vi "DriveExecuteTestFeedFoward.vi"(8 "error in (no error)":errorcluster) -> (0 "error out":errorcluster)   [LabVIEW 2020]
doc: "Execute and test/tune feed foward for Drive\n\nClosed control loop for drive\n\ninput: \n error in (cluster)\n\noutput:\n error out (cluster)"
uses:
  <vilib>/Rock Robotics/WPI/ThirdParty/Phoenix-LabVIEW/Motor Controller/Controls/CTRE_Phoenix_MotorControl_ControlMode.ctl
  <vilib>/Rock Robotics/WPI/ThirdParty/JAS_Junk/TrajLib/VI/Util_GetTime_U32.vi
  <vilib>/Rock Robotics/WPI/ThirdParty/JAS_Junk/TrajLib/SlewRateLimiter_New.vi
  <vilib>/Rock Robotics/WPI/ThirdParty/JAS_Junk/TrajLib/SlewRateLimiter_Reset.vi
  <vilib>/Rock Robotics/WPI/ThirdParty/JAS_Junk/TrajLib/SlewRateLimiter_Calculate.vi
  <vilib>/Rock Robotics/WPI/ThirdParty/JAS_Junk/TrajLib/SlewRateLimiter_SetRate.vi
  <vilib>/Rock Robotics/SystemInterfaces/Utilities/FPGA_UtilitiesRead LocalTime.vi
  <vilib>/Rock Robotics/WPI/ThirdParty/JAS_Junk/TrajLib/VI/Util_GetTime_U64.vi
  DriveGlobal.vi
  <vilib>/Rock Robotics/WPI/ThirdParty/Phoenix-LabVIEW/Motor Controller/Get/CTRE_Phoenix_MotorController_GetSelectedSensorData.vi
  <vilib>/Rock Robotics/WPI/ThirdParty/JAS_Junk/TrajLib/Trajectory_Library.lvlib
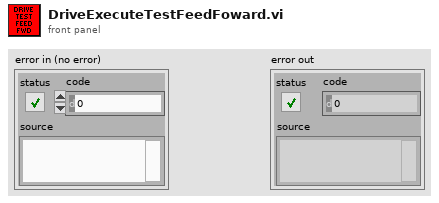
[diagram p1: front panel]
types:
  T1 = typedef "CTRE_Phoenix_MotorControl_ControlMode.ctl" = u16
  T2 = typedef "WPI_MotorControlDeviceRef.ctl" = cluster{"DeviceStatus":errorcluster, "Type":T3, "PWM":cluster{"PWM Channel":T4, "DeadBand":T5}, "CAN":cluster{"Device Number":u8, "SetOutput VI Ref":variant, "GetOutput VI Ref":variant, "Enable VI Ref":variant, "Disable VI Ref":variant, "Data":variant}, "Invert":bool, "DIO PWM":cluster{"PWM \"Enable\" Channel":T4, "DIOChannel":T6, "PWM Rate":dbl}}
  T3 = typedef "WPI_MotorControlType.ctl" = enum16{"PWM", "CAN", "DIO PWM"}
  T4 = typedef "FPGA_DIOPWMChannel.ctl" = enum8{"PWM 0", "PWM 1", "PWM 2", "PWM 3", "PWM 4", "PWM 5", "PWM 6", "PWM 7", "PWM 8", "PWM 9", "PWM MXP 0", "PWM MXP 1", "PWM MXP 2", "PWM MXP 3", "PWM MXP 4", "PWM MXP 5", "PWM MXP 6", "PWM MXP 7", "PWM MXP 8", "PWM MXP 9", "Invalid"}
  T5 = typedef "WPI_PWMDeadband.ctl" = cluster{"Name":string, "maxPositivePwm":i32, "minPositivePwm":i32, "centerPwm":i32, "maxNegativePwm":i32, "minNegativePwm":i32, "angularRange":u16}
  T6 = typedef "FPGA_DIOChannel.ctl" = enum8{"DIO 0", "DIO 1", "DIO 2", "DIO 3", "DIO 4", "DIO 5", "DIO 6", "DIO 7", "DIO 8", "DIO 9", "DIO MXP 0", "DIO MXP 1", "DIO MXP 2", "DIO MXP 3", "DIO MXP 4", "DIO MXP 5", "DIO MXP 6", "DIO MXP 7", "DIO MXP 8", "DIO MXP 9", "DIO MXP 10", "DIO MXP 11", "DIO MXP 12", "DIO MXP 13", "DIO MXP 14", "DIO MXP 15", "SPI Port CS1", "SPI Port CS2", "SPI Port CS3", "SPI Port MISO", "SPI Port MOSI", "Invalid"}
  T7 = typedef "ADIS16470 Device Reference.ctl" = cluster{"DevStatus":errorcluster, "Hardware Config":T8, "Calibration Complete":refnum<notifier>, "Status Reference":refnum<data-value>, "Data Reference":refnum<data-value>, "Sychronous Process VI":T11, "Cmd FIFO":refnum<k33>, "Source":T12, "Data FIFO":refnum<k33>, "Calibration Time (ms)":u32, "Data Reference":refnum<data-value>}
  T8 = typedef "ADIS16470 Hardware Configuration.ctl" = cluster{"SPI Clock Rate (Hz)":dbl, "IMU SPI Mode (3)":T9, "IMU Reset Pin":T6, "IMU SPI Bus":T10, "IMU Data Ready Pin":T6, "Stall Config":cluster{"Pow2BytesPerRead":u8, "StallTicks":u16, "CsToSclkTicks":u8}}
  T9 = typedef "WPI_SPIMode.ctl" = enum16{"Mode 0 (Clk Idle Low,Sample on Leading)", "Mode 1 (Clk Idle Low,Sample on Trailing)", "Mode 2 (Clk Idle High,Sample on Leading)", "Mode 3 (Clk Idle High,Sample on Trailing)"}
  T10 = typedef "spi_bus.ctl" = enum16{"SPI On-Board, CS0", "SPI On-Board, CS1", "SPI On-Board, CS2", "SPI On-Board, CS3", "SPI MXP", "Invalid"}
  T11 = typedef "ADIS16470 Process.ctl" = refnum<vi>
  T12 = typedef "FPGA_CounterEncoderSourceConvertionLVSourceType.ctl" = cluster{"DevStatus":errorcluster, "AnalogTriggerMode?":bool, "DigitalMode":cluster{"DIO Channel":T13}, "AnalogTriggerMode":cluster{"AnalogTriggerIndex":T14, "OutputType":T15}}
  T13 = typedef "FPGA_DIODigitalSourceChannel.ctl" = enum8{"DIO 0", "DIO 1", "DIO 2", "DIO 3", "DIO 4", "DIO 5", "DIO 6", "DIO 7", "DIO 8", "DIO 9", "DIO MXP 0", "DIO MXP 1", "DIO MXP 2", "DIO MXP 3", "DIO MXP 4", "DIO MXP 5", "DIO MXP 6", "DIO MXP 7", "DIO MXP 8", "DIO MXP 9", "DIO MXP 10", "DIO MXP 11", "DIO MXP 12", "DIO MXP 13", "DIO MXP 14", "DIO MXP 15", "SPI Port CS1", "SPI Port CS2", "SPI Port CS3", "SPI Port MISO", "SPI Port MOSI", "Disabled"}
  T14 = typedef "FPGA_AnalogTriggerIndex.ctl" = enum8{"Trig 0", "Trig 1", "Trig 2", "Trig 3", "Trig 4", "Trig 5", "Trig 6", "Trig 7", "Invalid"}
  T15 = typedef "FPGA_AnalogTriggerOutType.ctl" = enum16{"InWindow", "TriggerState", "Rising", "Falling"}
  T16 = typedef "ADIS16470 Data.ctl" = cluster{"XAngle":dbl, "YAngle":dbl, "ZAngle":dbl}
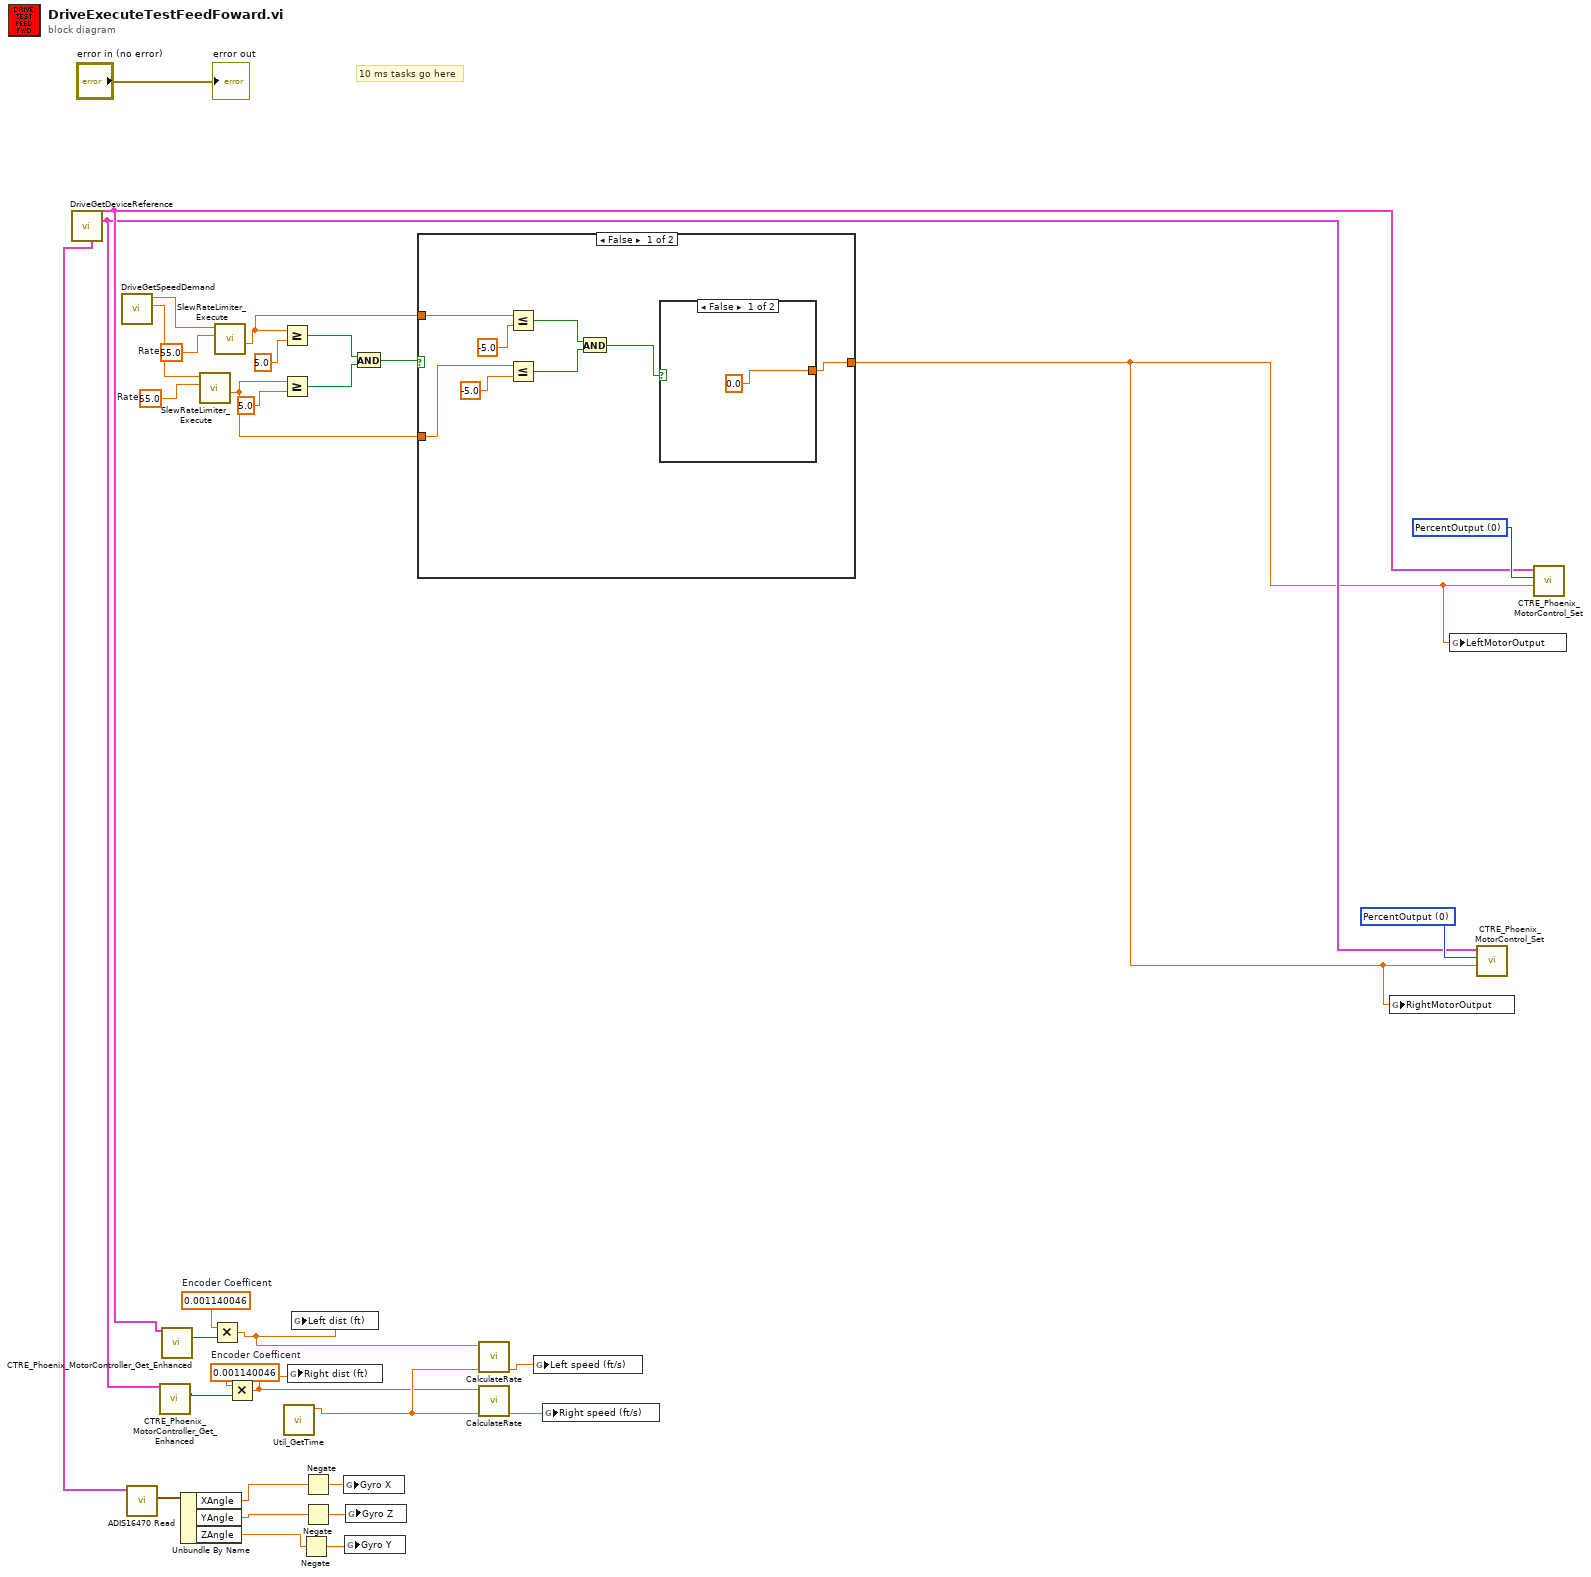
[diagram p0: block diagram]
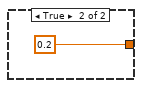
[diagram p2: hidden frame]
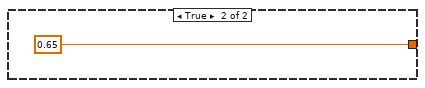
[diagram p3: hidden frame]
diagram:
  w16 = 55.0  # Rate
  w18 = 55.0  # Rate
  w21 = 0.001140046  # Encoder Coefficent
  w23 = 0.001140046  # Encoder Coefficent
  w33 = T1 0 items=["PercentOutput"=0, "Position"=1, "Velocity"=2, "Current"=3, "Follower"=5, "MotionProfile"=6, "MotionMagic"=7, "MotionProfileArc"=10, "Disabled"=15] ("Control Mode")
  w34 = T1 0 items=["PercentOutput"=0, "Position"=1, "Velocity"=2, "Current"=3, "Follower"=5, "MotionProfile"=6, "MotionMagic"=7, "MotionProfileArc"=10, "Disabled"=15] ("Control Mode")
  # "10 ms tasks go here"
  n1 = call "DriveGetDeviceReference.vi"() -> ("RightDriveTrain"=w25:T2, "LeftDriveTrain"=w26:T2, "Gryo"=w30:T7)  [unwired: 9 in]
  n2 = call "DriveGetSpeedDemand.vi"() -> ("RSpeedDemand (ft/s)"=w15:dbl, "LSpeedDemand (ft/s)"=w17:dbl)  [unwired: 10 in]
  n3 = call <vilib>:"ADIS16470 Read.vi"("ADIS16470DevRef"=w30) -> ("ADIS16470 Value"=w31:T16)  [unwired: 7 in, 3 out]
  n4 = call-poly <vilib>:"CTRE_Phoenix_MotorController_Get_Enhanced.vi"("PhoenixMotorControlDevRef"=w25) -> ("Position (Raw Sensor Units)"=w20:i32)  [unwired: 11 in, 3 out]
  n5 = call-poly <vilib>:"CTRE_Phoenix_MotorController_Get_Enhanced.vi"("PhoenixMotorControlDevRef"=w26) -> ("Position (Raw Sensor Units)"=w24:i32)  [unwired: 11 in, 3 out]
  n6 = Unbundle By Name(w31) -> ("XAngle"=w9:dbl, "YAngle"=w11:dbl, "ZAngle"=w10:dbl)
  n7 = call <vilib>:"SlewRateLimiter_Execute.vi"("PositiveRate"=w16, "Input"=w15) -> ("Output"=w1:dbl)  [unwired: 8 in, 1 out]
  n8 = Multiply(x=w23, y=w24) -> (x*y=w22:dbl)
  n9 = call <vilib>:"SlewRateLimiter_Execute.vi"("PositiveRate"=w18, "Input"=w17) -> ("Output"=w2:dbl)  [unwired: 8 in, 1 out]
  n10 = Multiply(x=w21, y=w20) -> (x*y=w19:dbl)
  n11 = Greater Or Equal?(x=w2, y=5.0) -> (x >= y?=w6:bool)
  n12 = Greater Or Equal?(x=w1, y=5.0) -> (x >= y?=w5:bool)
  n13 = call <vilib>:"Util_GetTime.vi"() -> ("FPGA_Time_Seconds"=w29:dbl)  [unwired: 9 in, 2 out]
  n14 = global write "DriveGlobal.vi" "Right dist (ft)"(w19) -> ()
  n15 = global write "DriveGlobal.vi" "Left dist (ft)"(w22) -> ()
  n16 = Negate(x=w10) -> (-x=w13:dbl)
  n17 = Negate(x=w9) -> (-x=w14:dbl)
  n18 = Negate(x=w11) -> (-x=w12:dbl)
  n19 = global write "DriveGlobal.vi" "Gyro X"(w14) -> ()
  n20 = global write "DriveGlobal.vi" "Gyro Y"(w13) -> ()
  n21 = global write "DriveGlobal.vi" "Gyro Z"(w12) -> ()
  n22 = And(x=w6, y=w5) -> (x .and. y?=w4:bool)
  n23 = case shown="False" w4 {
    tunnel: [w35 0.65] -> w3
    tunnel: w2 -> [w38 _]
    tunnel: w1 -> [w37 _]
    frame False {
      n24 = Less Or Equal?(x=w38, y=-5.0) -> (x <= y?=w41:bool)
      n25 = Less Or Equal?(x=w37, y=-5.0) -> (x <= y?=w42:bool)
      n26 = And(x=w41, y=w42) -> (x .and. y?=w36:bool)
      n27 = case shown="False" w36 {
        tunnel: [0.0 0.2] -> w35
        frame False {
        }
        frame True {
        }
      }
    }
    frame True {
    }
  }
  n28 = call "CalculateRate.vi"("Time (s)"=w29, "Distance (units)"=w22) -> ("Rate (units/s)"=w28:dbl)  [unwired: 9 in]
  n29 = call "CalculateRate.vi"("Time (s)"=w29, "Distance (units)"=w19) -> ("Rate (units/s)"=w27:dbl)  [unwired: 9 in]
  n30 = global write "DriveGlobal.vi" "Left speed (ft/s)"(w28) -> ()
  n31 = global write "DriveGlobal.vi" "Right speed (ft/s)"(w27) -> ()
  n32 = global write "DriveGlobal.vi" "RightMotorOutput"(w3) -> ()
  n33 = global write "DriveGlobal.vi" "LeftMotorOutput"(w3) -> ()
  n34 = call <vilib>:"CTRE_Phoenix_MotorControl_Set.vi"("Output"=w3, "Control Mode"=w33, "PhoenixMotorControlDevRef"=w25) -> ()  [unwired: 7 in, 2 out]
  n35 = call <vilib>:"CTRE_Phoenix_MotorControl_Set.vi"("Output"=w3, "Control Mode"=w34, "PhoenixMotorControlDevRef"=w26) -> ()  [unwired: 7 in, 2 out]
  "error out" <- "error in (no error)"
